vi "20220109_MultiFuncGen.vi"() -> ()   [LabVIEW 2021]
doc: "This example demonstrates how to generate a user-defined voltage using the analog output of a DAQ device."
uses:
  <vilib>/Utility/error.llb/DialogType.ctl
  <vilib>/DAQmx/write.llb/DAQmx Write (Analog 1D DBL NChan 1Samp).vi
  <vilib>/DAQmx/write.llb/DAQmx Write (Digital U8 1Chan 1Samp).vi
  <vilib>/DAQmx/create/channels.llb/DAQmx Create Channel (AO-Voltage-Basic).vi
  <vilib>/DAQmx/create/channels.llb/DAQmx Create Channel (DO-Digital Output).vi
  <vilib>/Utility/file.llb/Read Delimited Spreadsheet (DBL).vi
  <vilib>/DAQmx/miscellaneous.llb/DAQmx Fill In Error Info.vi
panel:
  in  "value":bool
  out "Waveform Chart":cluster{"Numeric":dbl, "Numeric":dbl}(graph)
  out "DIO":cluster{i16, i16, i16, i16, i16}(graph)
  in  "file path (dialog if empty)":path
  in  "DO":tag
  in  "AO":tag
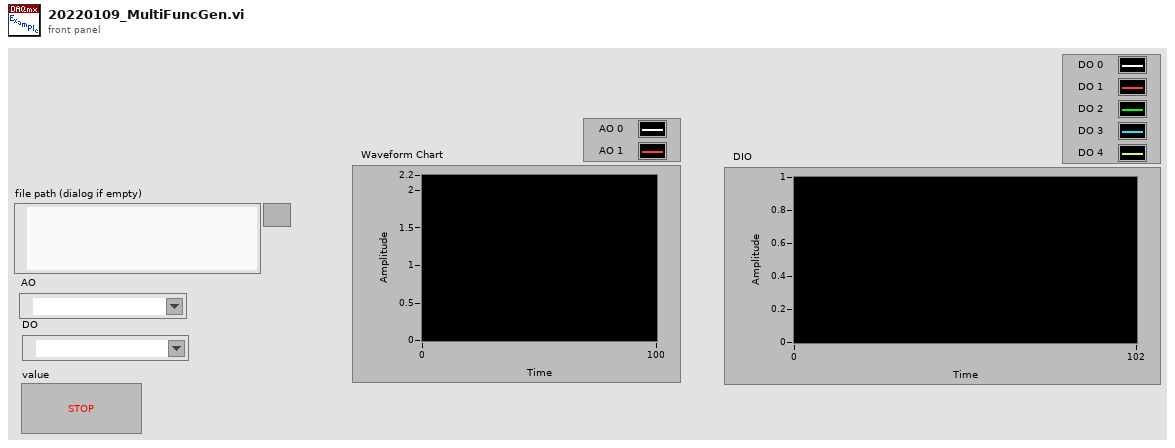
[diagram p1: front panel]
types:
  T1 = typedef "DialogType.ctl" = u16
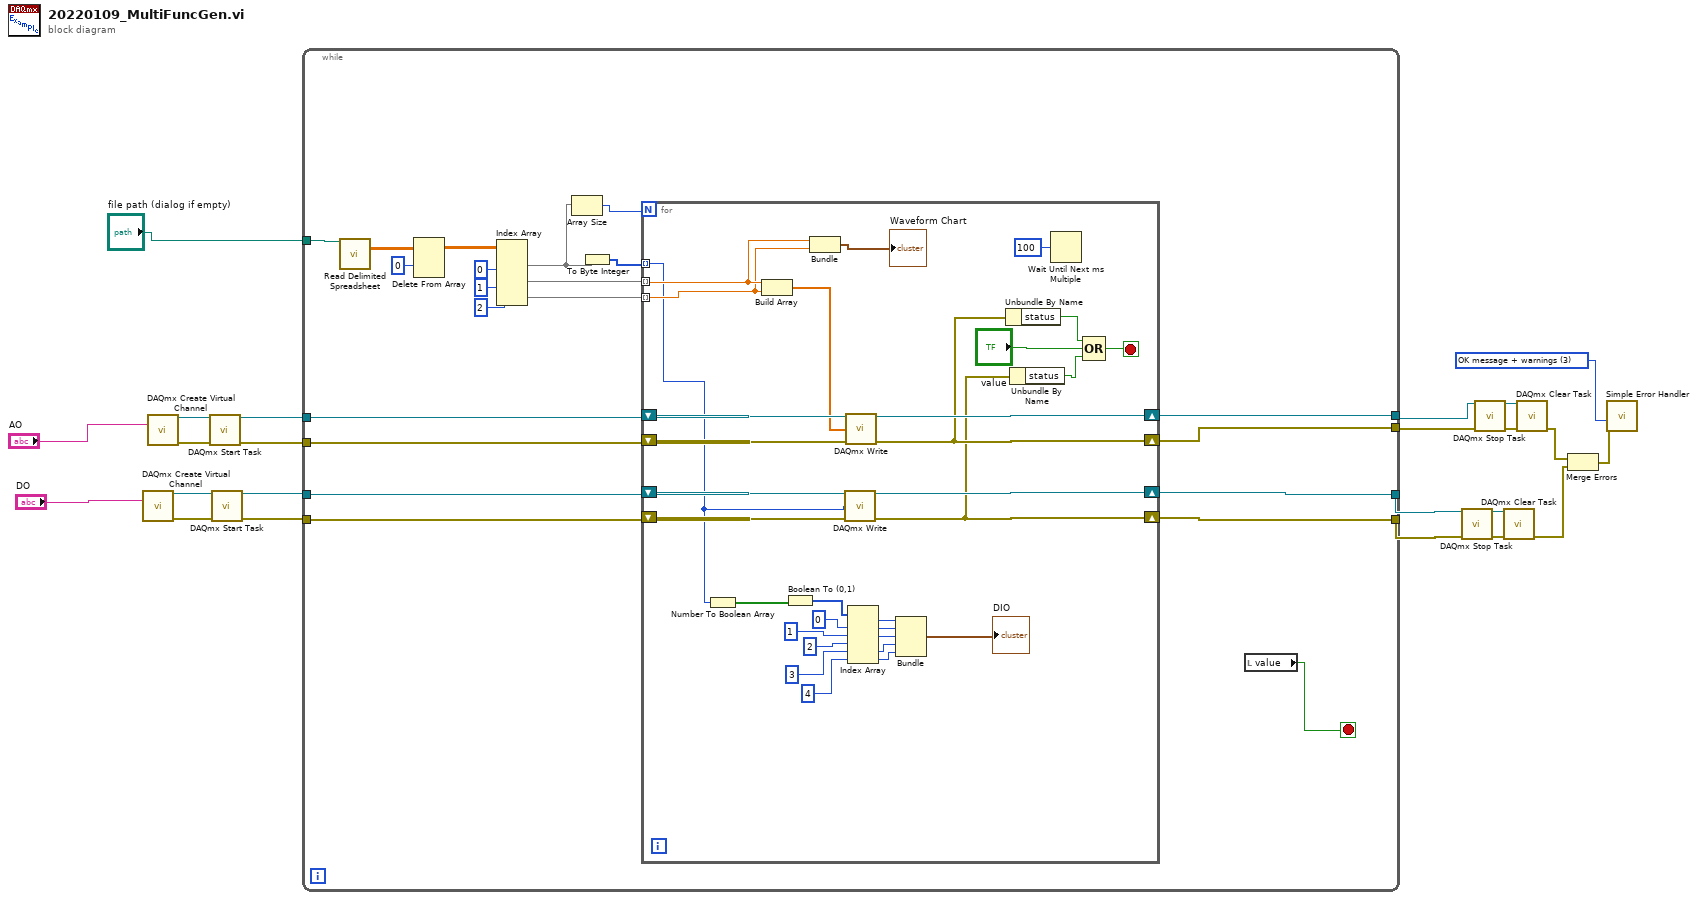
[diagram p0: block diagram]
diagram:
  w15 = T1 3 items=["no dialog", "OK message", "continue or stop message", "OK message + warnings", "continue/stop + warnings"] ("type of dialog (OK msg:1)")
  n1 = call-poly <vilib>:"DAQmx Create Virtual Channel.vi"("lines"="DO") -> ("task out"=w14:refnum<k21>, "error out"=w13:errorcluster)  [unwired: 13 in]
  n2 = call-poly <vilib>:"DAQmx Create Virtual Channel.vi"("physical channels"="AO") -> ("task out"=w23:refnum<k21>, "error out"=w22:errorcluster)  [unwired: 13 in]
  n3 = call <vilib>:"DAQmx Start Task.vi"("task/channels in"=w23, "error in"=w22) -> ("task out"=w21:refnum<k21>, "error out"=w20:errorcluster)  [unwired: 12 in]
  n4 = call <vilib>:"DAQmx Start Task.vi"("task/channels in"=w14, "error in"=w13) -> ("task out"=w12:refnum<k21>, "error out"=w11:errorcluster)  [unwired: 12 in]
  n5 = while {
    tunnel: w21 -> [w44]
    tunnel: w20 -> [w43]
    tunnel: [w41] -> w18
    tunnel: [w42] -> w19
    tunnel: w12 -> [w40]
    tunnel: w11 -> [w39]
    tunnel: [w38] -> w8
    tunnel: [w37] -> w7
    tunnel: "file path (dialog if empty)" -> [w29]
    stop <- w24 stop-if-true
    n6 = call-poly <vilib>:"Read Delimited Spreadsheet.vi"("file path (dialog if empty)"=w29) -> ("all rows"=w36:dbl[][])  [unwired: 9 in, 5 out]
    n7 = Delete From Array(array=w36, index (row)=0) -> (array with subset deleted=w34:dbl[][])  [unwired: 2 in, 1 out]
    n8 = Index Array(array=w34, index (col) #1=0 ("disabled index (col)"), index (col) #2=1 ("index (col)"), index (col) #3=2 ("index (col)")) -> (element #1=w30:dbl[], element #2=w26:dbl[], element #3=w25:dbl[])  [unwired: 3 in]
    n9 = Array Size(array=w30) -> (size(s)=w28:i32)
    n10 = To Byte Integer(number=w30) -> (8bit integer=w27:i8[])
    n11 = for {
      N: w28 -> [_]
      shift-right: [w73] -> w42
      shift-left: w44 -> [w75]
      shift-right: [w50] -> w41
      shift-left: w43 -> [w74]
      shift-right: [w70] -> w38
      shift-left: w40 -> [w72]
      shift-right: [w49] -> w37
      shift-left: w39 -> [w71]
      tunnel: w27 -> [w45] mode=indexing
      tunnel: w26 -> [w54] mode=indexing
      tunnel: w25 -> [w53] mode=indexing
      stop <- w47 stop-if-true
      n12 = Number To Boolean Array(number=w45) -> (Boolean array=w67:bool[])
      n13 = Build Array(w54, w53) -> (w68:dbl[])
      n14 = Boolean To (0,1)(Boolean=w67) -> (0, 1=w66:i16[])
      n15 = Bundle("Numeric"=w54, "Numeric"=w53) -> (→"Waveform Chart":cluster{"Numeric":dbl, "Numeric":dbl})  [unwired: 1 in]
      n16 = call-poly <vilib>:"DAQmx Write.vi"("task/channels in"=w72, "data"=w45, "error in"=w71) -> ("task out"=w70:refnum<k21>, "error out"=w49:errorcluster)  [unwired: 10 in, 1 out]
      n17 = call-poly <vilib>:"DAQmx Write.vi"("task/channels in"=w75, "data"=w68, "error in"=w74) -> ("task out"=w73:refnum<k21>, "error out"=w50:errorcluster)  [unwired: 10 in, 1 out]
      n18 = Index Array(array=w66, index #1=0 ("index"), index #2=1 ("index"), index #3=2 ("index"), index #4=3 ("index"), index #5=4 ("index")) -> (element #1=w60:i16, element #2=w59:i16, element #3=w58:i16, element #4=w57:i16, element #5=w56:i16)
      n19 = Bundle(w60, w59, w58, w57, w56) -> (→"DIO":cluster{i16, i16, i16, i16, i16})  [unwired: 1 in]
      n20 = Unbundle By Name(w50) -> ("status"=w48:bool)
      n21 = Unbundle By Name(w49) -> ("status"=w51:bool)
      n22 = Wait Until Next ms Multiple(millisecond multiple=u32 100) -> ()  [unwired: 1 out]
      n23 = Compound Arithmetic op=OR(w48, "value", w51) -> (w47:bool)
    }
    n24 = local read "value"() -> (w24:bool)
  }
  n25 = call <vilib>:"DAQmx Stop Task.vi"("task/channels in"=w8, "error in"=w7) -> ("task out"=w9:refnum<k21>, "error out"=w10:errorcluster)  [unwired: 12 in]
  n26 = call <vilib>:"DAQmx Stop Task.vi"("task/channels in"=w19, "error in"=w18) -> ("task out"=w17:refnum<k21>, "error out"=w16:errorcluster)  [unwired: 12 in]
  n27 = call <vilib>:"DAQmx Clear Task.vi"("task in"=w9, "error in"=w10) -> ("error out"=w2:errorcluster)  [unwired: 13 in]
  n28 = call <vilib>:"DAQmx Clear Task.vi"("task in"=w17, "error in"=w16) -> ("error out"=w3:errorcluster)  [unwired: 13 in]
  n29 = Merge Errors(w3, w2) -> (w4:errorcluster)
  n30 = call <vilib>:"Simple Error Handler.vi"("type of dialog (OK msg:1)"=w15, "error in (no error)"=w4) -> ()  [unwired: 3 in, 5 out]
